vi "main.vi"() -> ()   [LabVIEW 2015]
uses:
  resources/_reportList/ReportList.lvclass
  resources/_list/List.lvclass/List.ctl
  _ui/_list_UI/List_UI.lvclass/List_UI.ctl
  resources/_excel/Excel.lvclass
  resources/_list/List.lvclass
  _ui/_list_UI/List_UI.lvclass
panel:
  in  "Path":path
  in  "Table Control 2":string[][](table)
  in  "Table Control":string[][](table)
  in  "ExcelPath":path
  in  "RulesPath":path
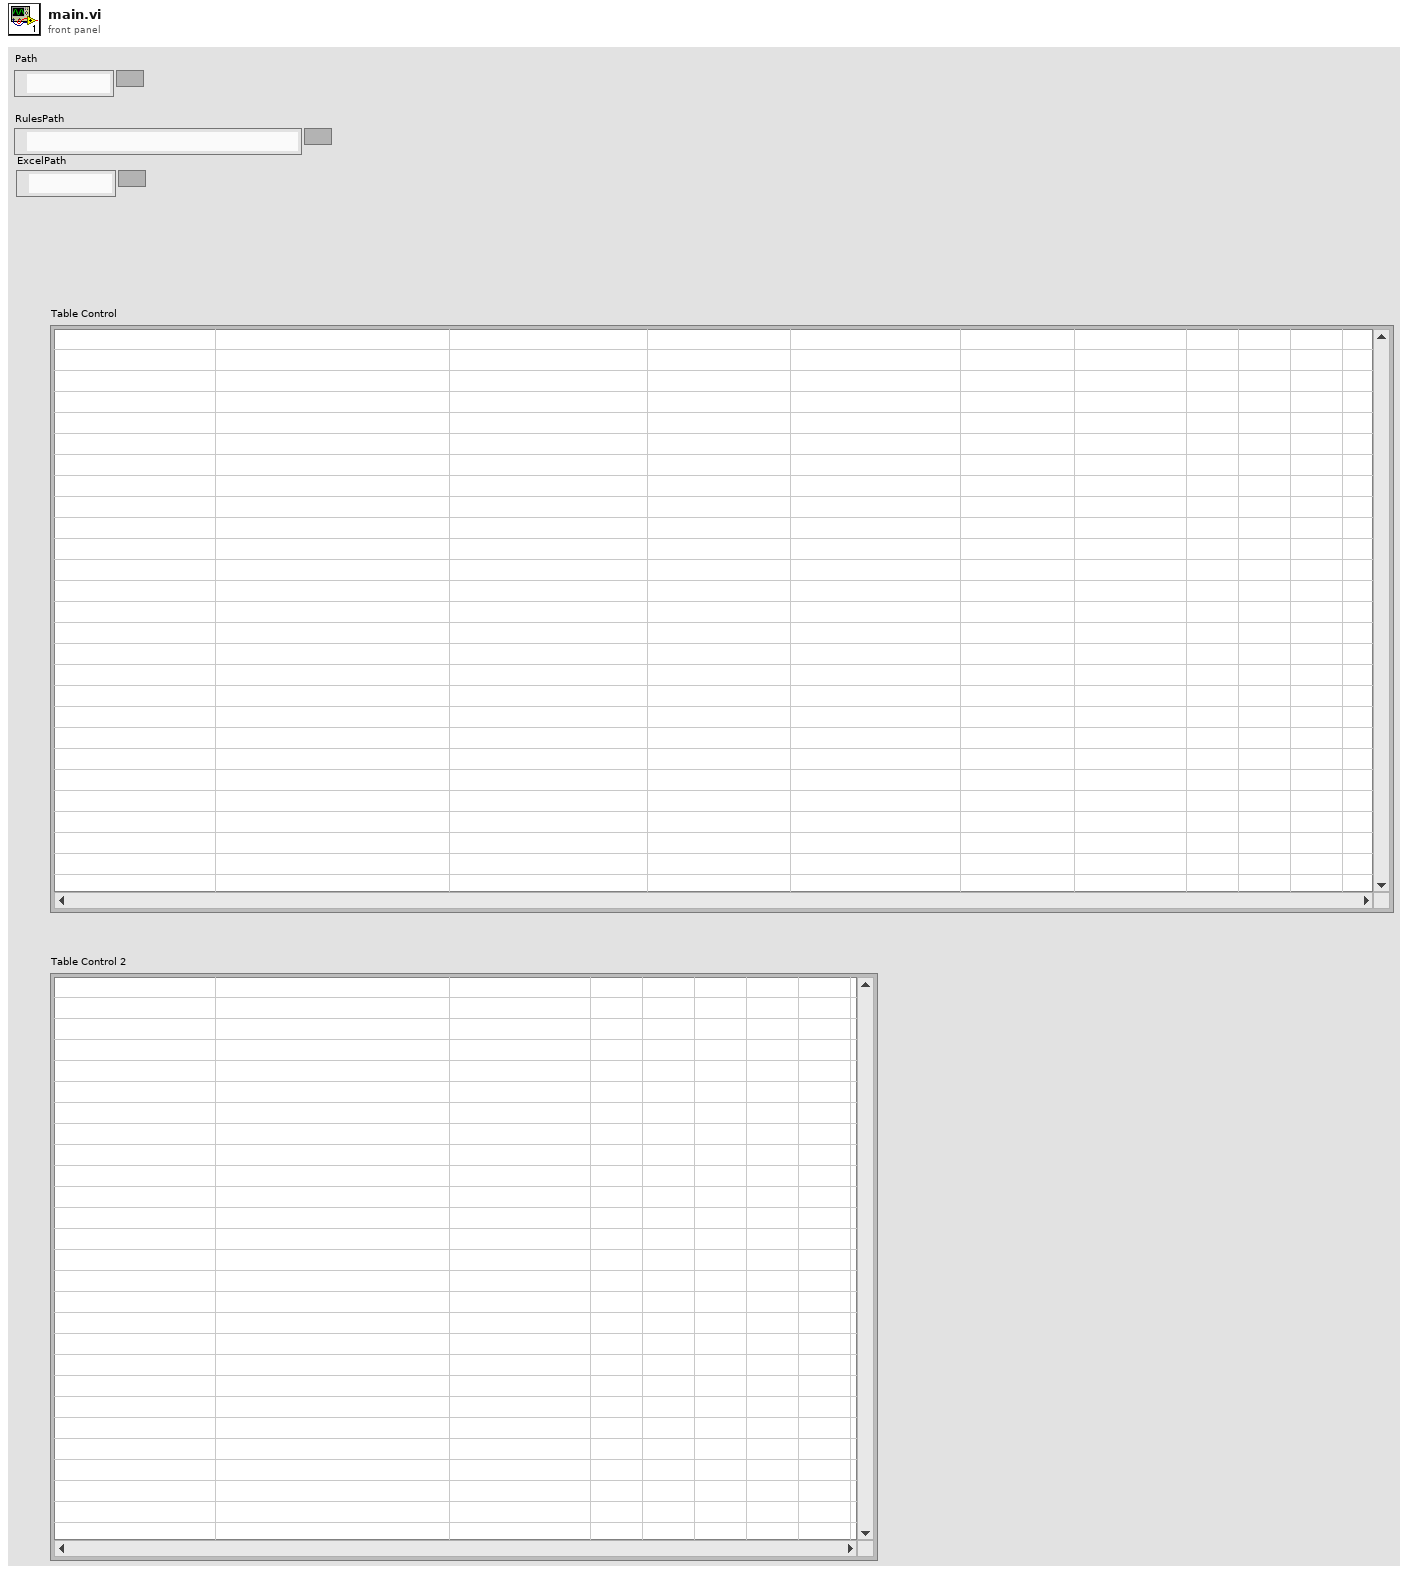
[diagram p1: front panel]
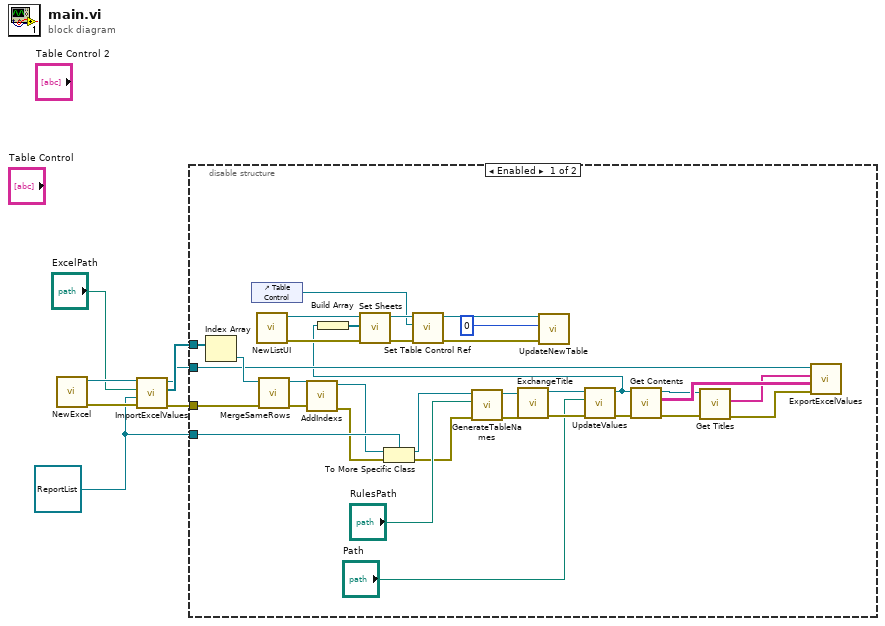
[diagram p0: block diagram]
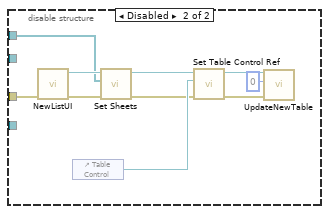
[diagram p2: hidden frame]
diagram:
  w2 = refnum<class "ReportList.lvclass"> refnum ("ReportList")
  n1 = call "NewExcel.vi"() -> ("error out"=w6:errorcluster, "Excel out"=w7:refnum<class "Excel.lvclass">)  [unwired: 10 in]
  n2 = call "ImportExcelValues.vi"("error in (no error)"=w6, "List In"=w2, "ExcelPath"="ExcelPath", "Excel in"=w7) -> ("error out"=w3:errorcluster, "Sheets"=w4:refnum<class "List.lvclass">[], "Excel out"=w1:refnum<class "Excel.lvclass">)  [unwired: 5 in]
  n3 = disable-structure shown="Enabled" {
    disable-tunnel: w4 -> [w40 w47]
    disable-tunnel: w3 -> [w38 w50]
    disable-tunnel: w2 -> [w37 _]
    disable-tunnel: w1 -> [w27 _]
    frame Enabled {
      n4 = Index Array(array=w40) -> (element=w39:refnum<class "List.lvclass">)  [unwired: 1 in]
      n5 = control-ref of="Table Control"() -> (w28:refnum<vi>)
      n6 = call "NewListUI.vi"() -> ("error out"=w34:errorcluster, "List_UI out"=w35:refnum<class "List_UI.lvclass">)  [unwired: 10 in]
      n7 = call "MergeSameRows.vi"("error in (no error)"=w38, "List in"=w39) -> ("error out"=w15:errorcluster, "List out"=w16:refnum<class "List.lvclass">)  [unwired: 8 in]
      n8 = call "AddIndexs.vi"("error in (no error)"=w15, "List in"=w16) -> ("error out"=w14:errorcluster, "List out"=w13:refnum<class "List.lvclass">)  [unwired: 8 in]
      n9 = To More Specific Class(target class=w37, reference=w13, error in=w14) -> (specific class reference=w21:refnum<class "ReportList.lvclass">, error out=w20:errorcluster)
      n10 = call "GenerateTableNames.vi"("error in (no error)"=w20, "Path"="RulesPath", "ReportList in"=w21) -> ("error out"=w19:errorcluster, "ReportList out"=w18:refnum<class "ReportList.lvclass">)  [unwired: 7 in]
      n11 = call "ExchangeTitle.vi"("error in (no error)"=w19, "List in"=w18) -> ("error out"=w11:errorcluster, "List out"=w12:refnum<class "ReportList.lvclass">)  [unwired: 8 in]
      n12 = call "UpdateValues.vi"("error in (no error)"=w11, "Path"="Path", "ReportList in"=w12) -> ("error out"=w10:errorcluster, "ReportList out"=w8:refnum<class "ReportList.lvclass">)  [unwired: 7 in]
      n13 = Build Array(w8) -> (w26:refnum<class "ReportList.lvclass">[])
      n14 = call "Set Sheets.vi"("error in (no error)"=w34, "Sheets"=w26, "List_UI in"=w35) -> ("error out"=w32:errorcluster, "List_UI out"=w33:refnum<class "List_UI.lvclass">)  [unwired: 7 in]
      n15 = call "Set Table Control Ref.vi"("error in (no error)"=w32, "Table Control"=w28, "List_UI in"=w33) -> ("error out"=w30:errorcluster, "List_UI out"=w31:refnum<class "List_UI.lvclass">)  [unwired: 7 in]
      n16 = call "UpdateNewTable.vi"("error in (no error)"=w30, "index"=0, "List_UI in"=w31) -> ()  [unwired: 7 in, 2 out]
      n17 = call "Get Contents.vi"("error in (no error)"=w10, "List in"=w8) -> ("error out"=w23:errorcluster, "Contents"=w25:string[][], "List out"=w24:refnum<class "ReportList.lvclass">)  [unwired: 7 in]
      n18 = call "Get Titles.vi"("error in (no error)"=w23, "List in"=w24) -> ("error out"=w17:errorcluster, "Titles"=w22:string[])  [unwired: 7 in, 1 out]
      n19 = call "ExportExcelValues.vi"("error in (no error)"=w17, "Contents"=w25, "Current Title"=w22, "Excel in"=w27) -> ()  [unwired: 6 in, 2 out]
    }
    frame Disabled {
      n20 = call "NewListUI.vi"("error in (no error)"=w50) -> ("error out"=w48:errorcluster, "List_UI out"=w49:refnum<class "List_UI.lvclass">)  [unwired: 9 in]
      n21 = control-ref of="Table Control"() -> (w46:refnum<vi>)
      n22 = call "Set Sheets.vi"("error in (no error)"=w48, "Sheets"=w47, "List_UI in"=w49) -> ("error out"=w44:errorcluster, "List_UI out"=w45:refnum<class "List_UI.lvclass">)  [unwired: 7 in]
      n23 = call "Set Table Control Ref.vi"("error in (no error)"=w44, "Table Control"=w46, "List_UI in"=w45) -> ("error out"=w42:errorcluster, "List_UI out"=w43:refnum<class "List_UI.lvclass">)  [unwired: 7 in]
      n24 = call "UpdateNewTable.vi"("error in (no error)"=w42, "index"=0, "List_UI in"=w43) -> ()  [unwired: 7 in, 2 out]
    }
  }
